vi "Disconnect Channels.vi"   [LabVIEW 2015, in "SLSC Switch.lvclass"]
uses:
  SLSC Switch.lvclass
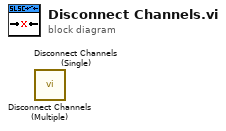
[diagram p0: block diagram]
diagram:
  n1 = call "Disconnect Channels (Multiple).vi"() -> ()  [unwired: 10 in, 2 out]
  n2 = call "Disconnect Channels (Single).vi"() -> ()  [unwired: 10 in, 2 out]
